vi "Array-Make String Unique.vi"(3 "Use parentheses":bool=TRUE, 4 "String":string, 5 "Strings":string[](array[string])) -> (1 "Unique String":string)   [LabVIEW 2020]
uses:
  <vilib>/regexp/Match Regular Expression.xnode
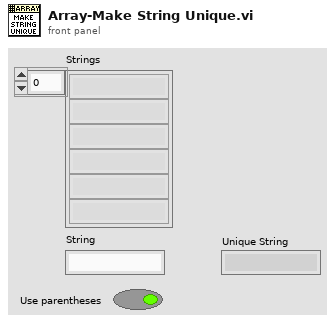
[diagram p1: front panel]
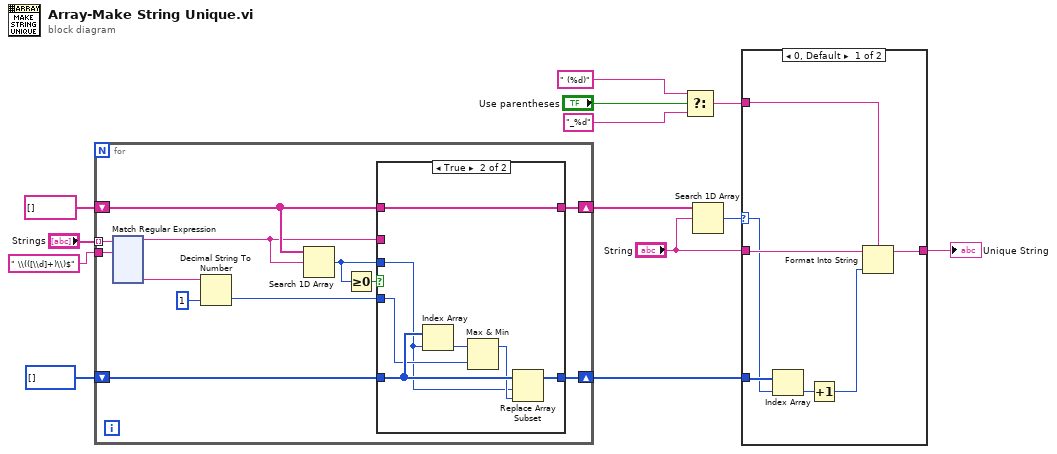
[diagram p0: block diagram]
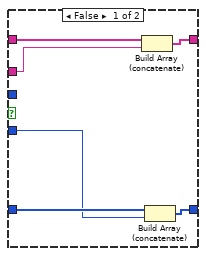
[diagram p3: hidden frame]
diagram:
  n1 = for {
    tunnel: "Strings" -> [w25] mode=indexing
    shift-right: [w16] -> w1
    shift-left: i32[] [] -> [w21]
    shift-right: [w17] -> w6
    shift-left: string[] [] -> [w22]
    tunnel: " \\(([\\d]+)\\)$" ("regular expression") -> [w24]
    n2 = xnode "Match Regular Expression"("input string"=w25, "regular expression"=w24) -> ("before match"=w20:string, "submatch 1"=w23:string)  [unwired: 4 in, 4 out]
    n3 = Decimal String To Number(string=w23, default (0L)=1 ("offset past number")) -> (number=w15:i32)  [unwired: 1 in, 1 out]
    n4 = Search 1D Array(1D array=w22, element=w20) -> (index of element=w18:i32)  [unwired: 1 in]
    n5 = Greater Or Equal To 0?(x=w18) -> (x >= 0?=w19:bool)
    n6 = case shown="True" w19 {
      tunnel: w22 -> [w31 w38]
      tunnel: w21 -> [w28 w37]
      tunnel: w20 -> [w29 _]
      tunnel: w15 -> [w26 w34]
      tunnel: w18 -> [_ w32]
      tunnel: [w30 w38] -> w17
      tunnel: [w27 w36] -> w16
      frame False {
        n7 = Build Array (concatenate)(w31, w29) -> (w30:string[])
        n8 = Build Array (concatenate)(w28, w26) -> (w27:i32[])
      }
      frame True {
        n9 = Index Array(array=w37, index=w32) -> (element=w35:i32)
        n10 = Max & Min(x=w35, y=w34) -> (max(x,y)=w33:i32)  [unwired: 1 out]
        n11 = Replace Array Subset(array=w37, new element=w33, index=w32) -> (w36:i32[])
      }
    }
  }
  n12 = Select(t=" (%d)" ("format string"), s="Use parentheses", f="_%d" ("format string")) -> (s? t:f=w2:string)
  n13 = Search 1D Array(1D array=w6, element="String") -> (index of element=w5:i32)  [unwired: 1 in]
  n14 = case shown="0, Default" w5 {
    selector: w5 -> [w157 _]
    tunnel: "String" -> [w161 w162]
    tunnel: [w159 w162] -> w3
    tunnel: w2 -> [w160 _]
    tunnel: w1 -> [w158 _]
    frame 0, Default {
      n15 = Index Array(array=w158, index=w157) -> (element=w156:i32)
      n16 = Increment(x=w156) -> (x+1=w155:i32)
      n17 = Format Into String(format string=w160, initial string=w161, w155) -> (resulting string=w159:string)  [unwired: 1 in, 1 out]
    }
    frame -1 {
    }
  }
  "Unique String" <- w3
